vi "update endtime.vi"(8 "error in (no error)":errorcluster, 10 "endtime":dbl, 11 "spec_dir":string) -> (0 "error out":errorcluster)   [LabVIEW 2019, in "libCheckpointUpdate.lvlib"]
doc: "void update_endtime(const char* spec_dir, double endtime);"
uses:
  libCheckpointUpdate.lvlib
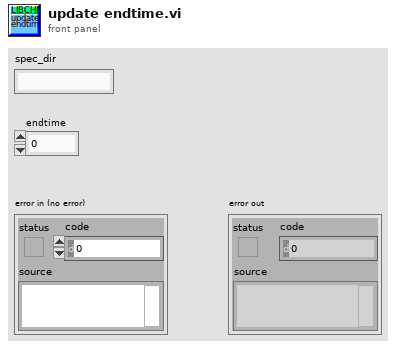
[diagram p1: front panel]
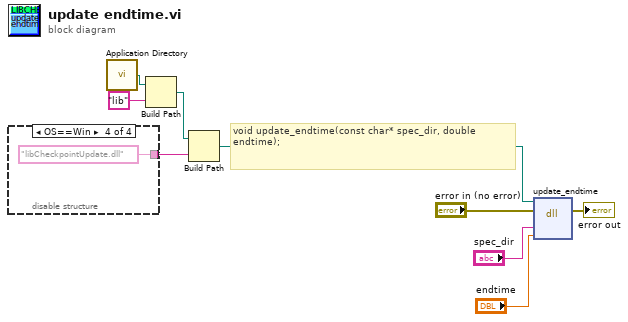
[diagram p0: block diagram]
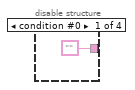
[diagram p2: hidden frame]
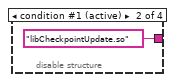
[diagram p3: hidden frame]
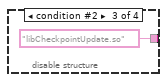
[diagram p4: hidden frame]
diagram:
  # "void update_endtime(const char* spec_dir, double endtime);"
  n1 = disable-structure shown="OS==Win" {
    disable-tunnel: ["" "libCheckpointUpdate.so" ("name or relative path") "libCheckpointUpdate.so" ("name or relative path") "libCheckpointUpdate.dll" ("name or relative path")] -> w1
    frame condition #0 {
    }
    frame condition #1 (active) {
    }
    frame condition #2 {
    }
    frame condition #3 {
    }
  }
  n2 = call <vilib>:"Application Directory.vi"() -> ("Application Directory"=w5:path)
  n3 = Build Path(base path=w5, name or relative path="lib") -> (appended path=w3:path)
  n4 = Build Path(base path=w3, name or relative path=w1) -> (appended path=w2:path)
  n5 = dll-call lib="home/paul/Schreibtisch/Biogas_plant_setup/LabView/lib/libCheckpointUpdate/libCheckpointUpdate.*" fn="update_endtime"(path in=w2, error in="error in (no error)", "spec_dir"="spec_dir", "endtime"="endtime") -> (error out=→"error out":errorcluster)  [unwired: 4 in, 1 out]
